vi "Destroy.vi"(8 "error in (no error)":errorcluster, 11 "MessageEvent":refnum<user-event>) -> (0 "error out":errorcluster)   [LabVIEW 2019, in "SLL Message.lvlib"]
uses:
  SLL Message.lvlib
  Typedefs/Message.ctl
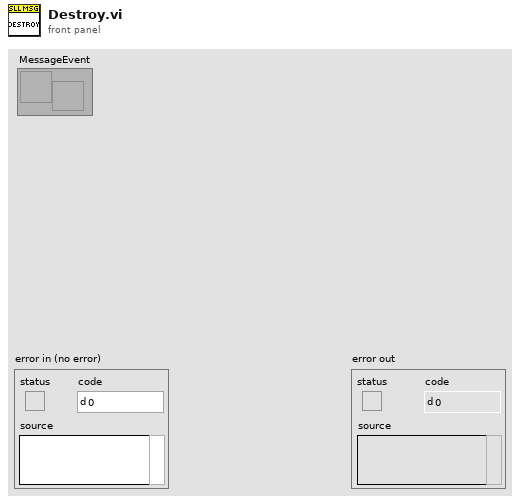
[diagram p1: front panel]
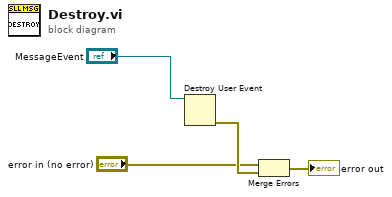
[diagram p0: block diagram]
diagram:
  n1 = Destroy User Event(user event="MessageEvent") -> (error out=w2:errorcluster)  [unwired: 1 in]
  n2 = Merge Errors("error in (no error)", w2) -> (→"error out":errorcluster)
